vi "VI Tree.vi"   [LabVIEW 2012, in "Phidget LCD.lvlib"]
doc: "${LCD:VITreeHeader}"
uses:
  <instrlib>/Phidgets/Phidget LCD/Phidget LCD.lvlib
  <instrlib>/Phidgets/Phidget LCD/Public/LCDStart.vi
  <instrlib>/Phidgets/Phidget LCD/Public/LCDOpen.vi
  <instrlib>/Phidgets/Phidget LCD/Public/LCDClose.vi
panel:
  # "(c) 2015 Phidgets Inc..  ALL RIGHTS RESERVED."
  # "SEE DIAGRAM\nFOR VI TREE."
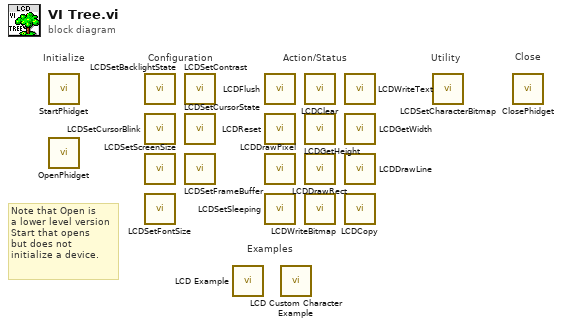
[diagram p0: block diagram]
diagram:
  # "Note that Open is\na lower level version\nStart that opens\nbut does not \ninitialize a device."
  # "Examples"
  # "Configuration"
  # "Utility"
  # "Action/Status"
  # "Close"
  # "Initialize"
  n1 = call-poly <instrlib>:"StartPhidget.vi"() -> ()  [unwired: 12 in, 4 out]
  n2 = call-poly <instrlib>:"OpenPhidget.vi"() -> ()  [unwired: 8 in, 4 out]
  n3 = call <instrlib>:"LCDSetBacklightState.vi"() -> ()  [unwired: 9 in, 2 out]
  n4 = call <instrlib>:"LCDSetCursorBlink.vi"() -> ()  [unwired: 9 in, 2 out]
  n5 = call <instrlib>:"LCDSetScreenSize.vi"() -> ()  [unwired: 9 in, 2 out]
  n6 = call <instrlib>:"LCDSetFontSize.vi"() -> ()  [unwired: 10 in, 2 out]
  n7 = call <instrlib>:"LCDSetContrast.vi"() -> ()  [unwired: 9 in, 2 out]
  n8 = call <instrlib>:"LCDSetCursorState.vi"() -> ()  [unwired: 9 in, 2 out]
  n9 = call <instrlib>:"LCDSetFrameBuffer.vi"() -> ()  [unwired: 10 in, 2 out]
  n10 = call <instrlib>:"LCD Example.vi"() -> ()  [unwired: 12 in]
  n11 = call <instrlib>:"LCDFlush.vi"() -> ()  [unwired: 9 in, 2 out]
  n12 = call <instrlib>:"LCDReset.vi"() -> ()  [unwired: 9 in, 2 out]
  n13 = call <instrlib>:"LCDDrawPixel.vi"() -> ()  [unwired: 10 in, 2 out]
  n14 = call <instrlib>:"LCDSetSleeping.vi"() -> ()  [unwired: 10 in, 2 out]
  n15 = call <instrlib>:"LCD Custom Character Example.vi"() -> ()  [unwired: 12 in]
  n16 = call <instrlib>:"LCDClear.vi"() -> ()  [unwired: 9 in, 2 out]
  n17 = call <instrlib>:"LCDGetHeight.vi"() -> ()  [unwired: 9 in, 3 out]
  n18 = call <instrlib>:"LCDDrawRect.vi"() -> ()  [unwired: 10 in, 2 out]
  n19 = call <instrlib>:"LCDWriteBitmap.vi"() -> ()  [unwired: 10 in, 2 out]
  n20 = call <instrlib>:"LCDWriteText.vi"() -> ()  [unwired: 14 in, 2 out]
  n21 = call <instrlib>:"LCDGetWidth.vi"() -> ()  [unwired: 9 in, 3 out]
  n22 = call <instrlib>:"LCDDrawLine.vi"() -> ()  [unwired: 10 in, 2 out]
  n23 = call <instrlib>:"LCDCopy.vi"() -> ()  [unwired: 18 in, 2 out]
  n24 = call <instrlib>:"LCDSetCharacterBitmap.vi"() -> ()  [unwired: 10 in, 2 out]
  n25 = call-poly <instrlib>:"ClosePhidget.vi"() -> ()  [unwired: 11 in, 1 out]
